vi "VI Tree.vi"   [LabVIEW 2018, in "QueueTimer.lvlib"]
doc: "Queue timer library contains the following:\n- <b>Examples</b> - Example VIs\n- <b>API</b> - Top-level VIs\n- <b>SubVIs</b> - Low-level VIs"
uses:
  QueueTimer.lvlib
  TypeDefs/Timer.ctl
types:
  T1 = typedef "QueueTimer.lvlib/Timer.ctl" = cluster{"Delay":i32, "Start":bool, "Ticks":u32}
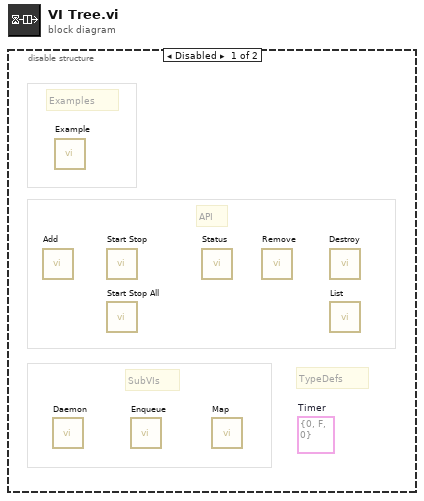
[diagram p0: block diagram]
diagram:
  n1 = disable-structure shown="Disabled" {
    frame Disabled {
      (unwired) T1 {"Delay"=0, "Start"=FALSE, "Ticks"=0}  # Timer
      # "Examples"
      # "SubVIs"
      # "TypeDefs"
      # "API"
      n2 = call "Add.vi"() -> ()  [unwired: 9 in, 3 out]
      n3 = call "Daemon.vi"() -> ()  [unwired: 12 in]
      n4 = call "Example.vi"() -> ()  [unwired: 12 in]
      n5 = call "Start Stop.vi"() -> ()  [unwired: 10 in, 2 out]
      n6 = call "Start Stop All.vi"() -> ()  [unwired: 9 in, 3 out]
      n7 = call "Enqueue.vi"() -> ()  [unwired: 10 in, 2 out]
      n8 = call "Status.vi"() -> ()  [unwired: 6 in, 6 out]
      n9 = call "Map.vi"() -> ()  [unwired: 10 in, 2 out]
      n10 = call "Remove.vi"() -> ()  [unwired: 9 in, 3 out]
      n11 = call "Destroy.vi"() -> ()  [unwired: 9 in, 3 out]
      n12 = call "List.vi"() -> ()  [unwired: 10 in, 2 out]
    }
    frame Enabled {
    }
  }
